vi "GetToteSequence.vi"() -> ()   [LabVIEW 2014]
panel:
  out "Transverse Wheels 3":bool
  out "Transverse Wheels":bool
  in  "Tusks":bool
  in  "Transverse Wheels":bool
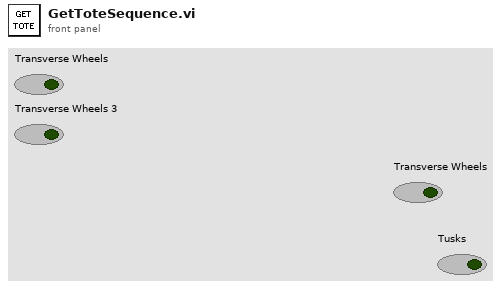
[diagram p1: front panel]
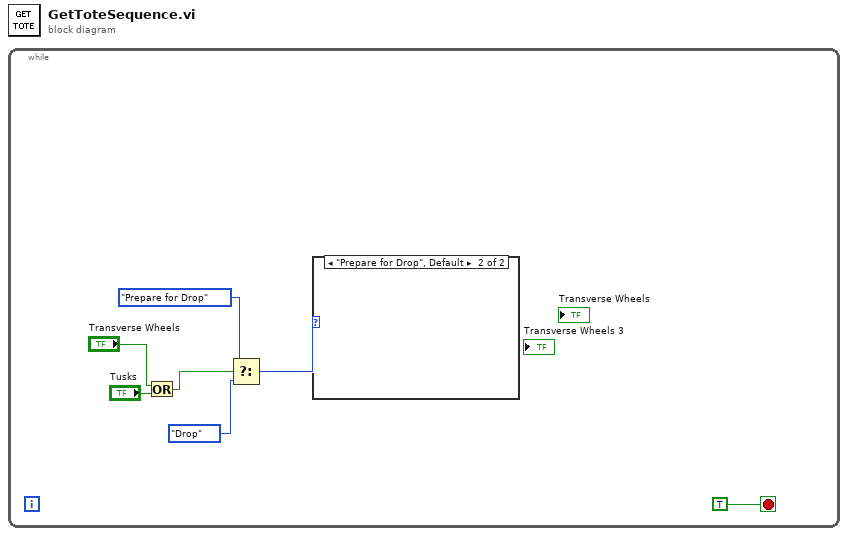
[diagram p0: block diagram]
diagram:
  n1 = while {
    stop <- TRUE stop-if-true
    n2 = Or(x="Transverse Wheels", y="Tusks") -> (x .or. y?=w4:bool)
    n3 = Select(t=enum16{"Drop", "Prepare for Drop"}."Prepare for Drop", s=w4, f=enum16{"Drop", "Prepare for Drop"}."Drop") -> (s? t:f=w1:enum16{"Drop", "Prepare for Drop"})
    n4 = case shown="\"Prepare for Drop\", Default" w1 {
      frame "Drop" {
      }
      frame "Prepare for Drop", Default {
      }
    }
  }
